vi "New.vi"(6 "Creator":refnum<class "Msg Type Strategy.lvclass">, 8 "Creator Alias":string, 9 "Self":refnum<class "Msg Type Strategy.lvclass">, 10 "Self Alias":string) -> (0 "error out":errorcluster, 2 "Addresses DVR":refnum<data-value>)   [LabVIEW 2021, in "jettl.lvlib" / "Addresses.lvlib"]
uses:
  Addresses.lvlib
  Addresses/Addresses.lvclass
  Msg Type Strategy/Msg Type Strategy/Msg Type Strategy.lvclass
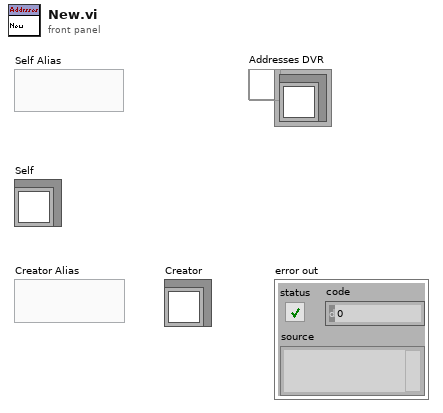
[diagram p1: front panel]
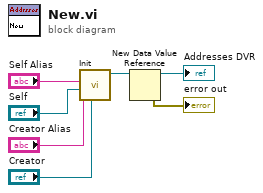
[diagram p0: block diagram]
diagram:
  n1 = call "Init.vi"("Creator"="Creator", "Creator Alias"="Creator Alias", "Self"="Self", "Self Alias"="Self Alias") -> ("Addresses out"=w5:refnum<class "Addresses.lvclass">)  [unwired: 7 in]
  n2 = New Data Value Reference(data value=w5) -> (data value reference=→"Addresses DVR":refnum<data-value>, error out=→"error out":errorcluster)  [unwired: 1 in]
